vi "MD5_evaluation.vi"(9 "ServerInfo":T1={"nonce from server"="dcd98b7102dd2f0e8b11d0f600bfb0c093", "qop "="auth"}, 11 "ClientInfo":T2={"username"="Mufasa", "realm"="testrealm@host.com", "password"="Circle Of Life", "method"="GET", "digestURI"="/dir/index.html"}) -> (1 "response":string, 2 "HA2":string, 3 "HA1":string, 5 "cnonce of client":string, 7 "RequestCounter":string)   [LabVIEW 2016]
uses:
  Program Files/National Instruments/LabVIEW 2016/user.lib/_OpenG.lib/md5/md5.llb/MD5 Message Digest (Hexadecimal String)__ogtk.vi
panel:
  out "MD5 Hash?":bool
  out "concatenated string":string
  # "(quality of protection code) from server"
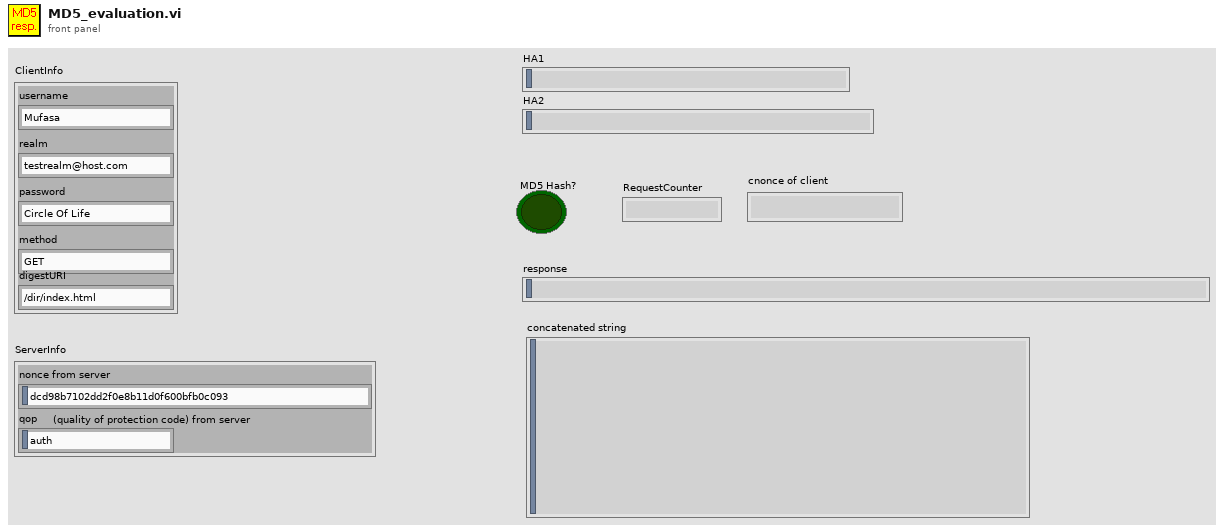
[diagram p1: front panel]
types:
  T1 = cluster{"nonce from server":string, "qop ":string}
  T2 = cluster{"username":string, "realm":string, "password":string, "method":string, "digestURI":string}
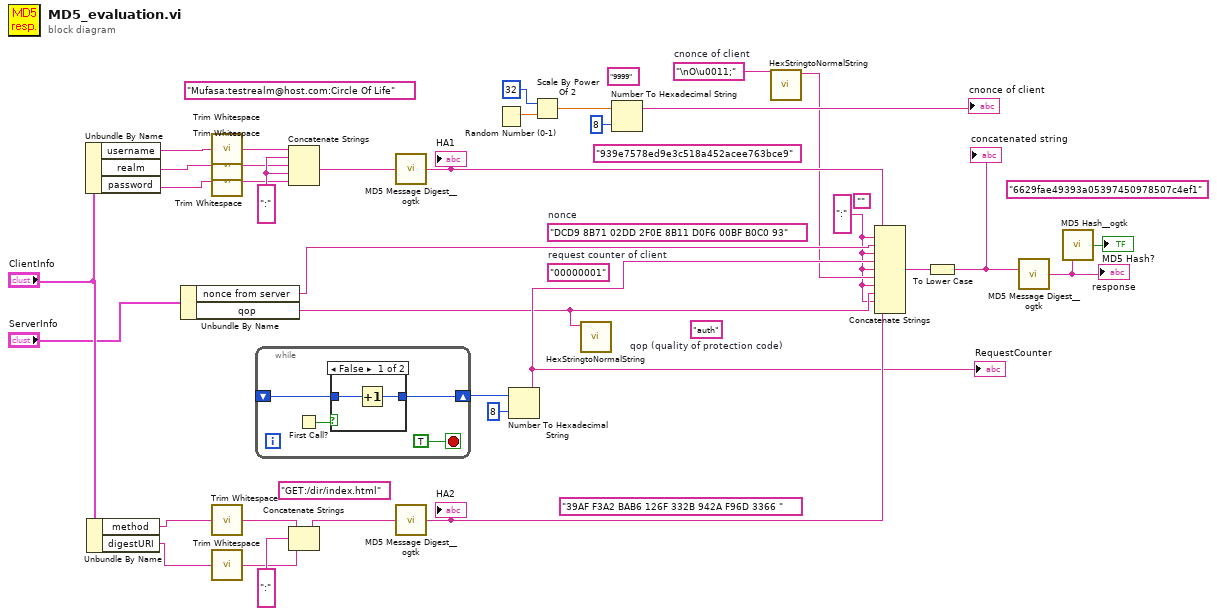
[diagram p0: block diagram]
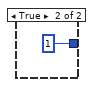
[diagram p2: hidden frame]
diagram:
  (unwired) "6629fae49393a05397450978507c4ef1" ("MD5 Message Digest 2")
  (unwired) "9999" ("string in (not encoded)")
  w30 = ":" ("string")
  (unwired) ""
  (unwired) "auth"  # qop (quality of protection code)
  w5 = "\nO\u0011;"  # cnonce of client
  (unwired) "00000001"  # request counter of client
  w2 = ":" ("string")
  (unwired) "DCD9 8B71 02DD 2F0E 8B11 D0F6 00BF B0C0 93"  # nonce
  (unwired) "39AF F3A2 BAB6 126F 332B 942A F96D 3366 " ("MD5 Message Digest 2")
  (unwired) "GET:/dir/index.html" ("Message")
  (unwired) "939e7578ed9e3c518a452acee763bce9" ("MD5 Message Digest")
  (unwired) "Mufasa:testrealm@host.com:Circle Of Life" ("Message")
  n1 = Unbundle By Name("ClientInfo") -> ("username"=w23:string, "realm"=w22:string, "password"=w21:string)
  n2 = Unbundle By Name("ClientInfo") -> ("method"=w19:string, "digestURI"=w18:string)
  n3 = Unbundle By Name("ServerInfo") -> ("nonce from server"=w16:string, "qop"=w3:string)
  n4 = call <vilib>:"Trim Whitespace.vi"("string"=w23) -> ("trimmed string"=w28:string)  [unwired: 1 in]
  n5 = call <vilib>:"Trim Whitespace.vi"("string"=w22) -> ("trimmed string"=w27:string)  [unwired: 1 in]
  n6 = call <vilib>:"Trim Whitespace.vi"("string"=w21) -> ("trimmed string"=w26:string)  [unwired: 1 in]
  n7 = call <vilib>:"Trim Whitespace.vi"("string"=w19) -> ("trimmed string"=w25:string)  [unwired: 1 in]
  n8 = call <vilib>:"Trim Whitespace.vi"("string"=w18) -> ("trimmed string"=w24:string)  [unwired: 1 in]
  n9 = while {
    shift-right: [w37] -> w7
    shift-left: _ -> [w36]
    stop <- TRUE stop-if-true
    n10 = First Call?() -> (First Call?: T/F=w38:bool)
    n11 = case shown="False" w38 {
      tunnel: [w40 1] -> w37
      tunnel: w36 -> [w41 _]
      frame False {
        n12 = Increment(x=w41) -> (x+1=w40:i32)
      }
      frame True {
      }
    }
  }
  n13 = Concatenate Strings(w28, w30, w27, w30, w26) -> (w29:string)
  n14 = Concatenate Strings(w25, ":" ("string"), w24) -> (w31:string)
  n15 = call-poly "MD5 Message Digest__ogtk.vi"("Message"=w29) -> ("MD5 Message Digest"=w35:string)
  "HA1" <- w35
  n16 = call-poly "MD5 Message Digest__ogtk.vi"("Message"=w31) -> ("MD5 Message Digest"=w34:string)
  "HA2" <- w34
  n17 = Random Number (0-1)() -> (number: 0 to 1=w13:dbl)
  n18 = Number To Hexadecimal String(1:i16 8 ("width (-)"), 2:w7) -> (0:w6:string)
  "RequestCounter" <- w6
  n19 = Scale By Power Of 2(n=i16 32, x=w13) -> (x*2^n=w11:dbl)
  n20 = call "HexStringtoNormalString.vi"("String in (hex)."=w3) -> ()  [unwired: 10 in, 1 out]
  n21 = Number To Hexadecimal String(1:i16 8 ("width (-)"), 2:w11) -> (0:→"cnonce of client":string)
  n22 = call "HexStringtoNormalString.vi"("String in (hex)."=w5) -> ("String out (normal)"=w4:string)  [unwired: 10 in]
  n23 = Concatenate Strings(w35, w2, w16, w2, w6, w2, w4, w2, w3, w2, w34) -> (w33:string)
  n24 = To Lower Case(string=w33) -> (all lower case string=w1:string)
  "concatenated string" <- w1
  n25 = call-poly "MD5 Message Digest__ogtk.vi"("Message"=w1) -> ("MD5 Message Digest"=w15:string)
  "response" <- w15
  n26 = call "MD5 Hash__ogtk.vi"("Input String"=w15) -> ("MD5 Hash?"=→"MD5 Hash?":bool)  [unwired: 3 in]
